vi "Update FCR parameters -- subVI.vi"(8 "error in (no error)":errorcluster, 9 "Velocity":dbl, 10 "Aceleration":dbl, 11 "FCR Mod ID":i32) -> (0 "error out":errorcluster)   [LabVIEW 2020]
uses:
  Newport_FCR100/Libraries/FCR100/FCR100.lvlib
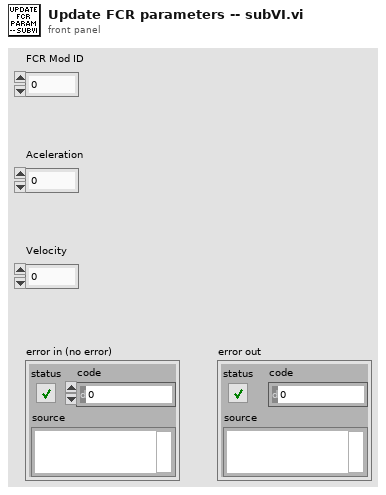
[diagram p1: front panel]
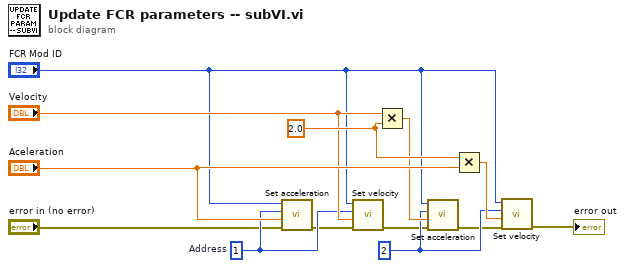
[diagram p0: block diagram]
diagram:
  w12 = 2.0 ("y")
  w8 = u8 2 ("Address")
  w3 = u8 1  # Address
  n1 = call "Set acceleration.vi"("error in"="error in (no error)", "Acceleration"="Aceleration", "Address"=w3, "Module ID"="FCR Mod ID") -> ("error out"=w2:errorcluster)  [unwired: 7 in]
  n2 = call "Set velocity.vi"("error in"=w2, "Velocity"="Velocity", "Address"=w3, "Module ID"="FCR Mod ID") -> ("error out"=w4:errorcluster)  [unwired: 7 in]
  n3 = Multiply(x="Velocity", y=w12) -> (x*y=w10:dbl)
  n4 = call "Set acceleration.vi"("error in"=w4, "Acceleration"=w10, "Address"=w8, "Module ID"="FCR Mod ID") -> ("error out"=w5:errorcluster)  [unwired: 7 in]
  n5 = Multiply(x=w12, y="Aceleration") -> (x*y=w13:dbl)
  n6 = call "Set velocity.vi"("error in"=w5, "Velocity"=w13, "Address"=w8, "Module ID"="FCR Mod ID") -> ("error out"=→"error out":errorcluster)  [unwired: 7 in]
